vi "plotUpdate.vi"(6 "robotPosition":T2, 8 "plotPoints":cluster{dbl, dbl}[](array[cluster]), 11 "Image":T1) -> (3 "imageOut":T1)   [LabVIEW 2015]
uses:
  <vilib>/vision/Image Controls.llb/IMAQ Image.ctl
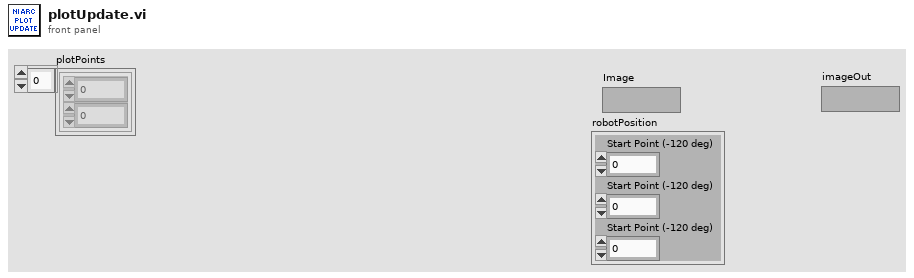
[diagram p1: front panel]
types:
  T1 = typedef "IMAQ Image.ctl" = refnum<image>
  T2 = cluster{"Start Point (-120 deg)":dbl, "Start Point (-120 deg)":dbl, "Start Point (-120 deg)":dbl}
  T3 = cluster{"Start Point (-120 deg)":dbl, "Start Point (-120 deg)":dbl}
  T4 = cluster{"Start Point (-120 deg)":dbl, "Start Point (-120 deg)":dbl, "Start Point (-120 deg)":dbl, "Start Point (-120 deg)":dbl}
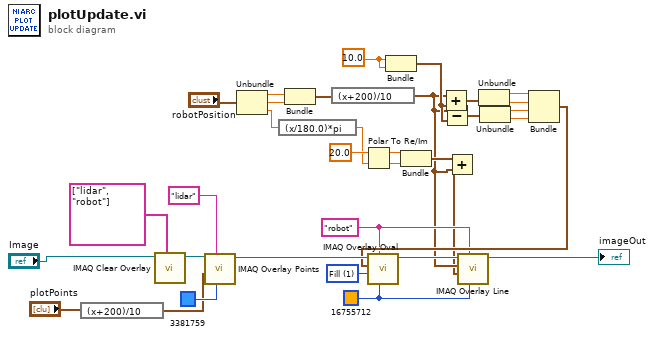
[diagram p0: block diagram]
diagram:
  w13 = u32 1 items=["Frame", "Fill"] ("Drawing Mode (Frame)")
  w22 = 10.0 ("Start Point (-120 deg)")
  w10 = "robot" ("Group")
  w11 = u32 16755712 ("Color")
  n1 = expression code="(x+200)/10"("plotPoints") -> (w30:cluster{dbl, dbl}[])
  n2 = call "IMAQ Clear Overlay"("Groups"=string[] ["lidar", "robot"], "Image"="Image") -> ("Image Out"=w32:T1)  [unwired: 8 in, 1 out]
  n3 = call "IMAQ Overlay Points"("Color"=u32 3381759, "Group"="lidar", "Array of Points"=w30, "Image"=w32) -> ("Image Out"=w27:T1)  [unwired: 6 in, 1 out]
  n4 = Unbundle("robotPosition") -> ("Start Point (-120 deg)"=w25:dbl, "Start Point (-120 deg)"=w24:dbl, "Start Point (-120 deg)"=w8:dbl)
  n5 = expression code="(x/180.0)*pi" ("degrees to radians")(w8) -> (w7:dbl)
  n6 = Bundle("Start Point (-120 deg)"=w25, "Start Point (-120 deg)"=w24) -> (w23:T3)  [unwired: 1 in]
  n7 = expression code="(x+200)/10"(w23) -> (w3:T3)
  n8 = Polar To Re/Im(2:w7, 3:20.0 ("r")) -> (0:w6:dbl, 1:w5:dbl)
  n9 = Bundle("Start Point (-120 deg)"=w22, "Start Point (-120 deg)"=w22) -> (w21:T3)  [unwired: 1 in]
  n10 = Bundle(w5, w6) -> (w4:cluster{dbl, dbl})  [unwired: 1 in]
  n11 = Add(x=w3, y=w21) -> (x+y=w20:T3)
  n12 = Subtract(x=w3, y=w21) -> (x-y=w19:T3)
  n13 = Add(x=w4, y=w3) -> (x+y=w2:cluster{dbl, dbl})
  n14 = Unbundle(w20) -> ("Start Point (-120 deg)"=w18:dbl, "Start Point (-120 deg)"=w17:dbl)
  n15 = Unbundle(w19) -> ("Start Point (-120 deg)"=w16:dbl, "Start Point (-120 deg)"=w15:dbl)
  n16 = Bundle("Start Point (-120 deg)"=w18, "Start Point (-120 deg)"=w17, "Start Point (-120 deg)"=w16, "Start Point (-120 deg)"=w15) -> (w14:T4)  [unwired: 1 in]
  n17 = call "IMAQ Overlay Oval"("Color"=w11, "Group"=w10, "Drawing Mode (Frame)"=w13, "Bounding Rectangle"=w14, "Image"=w27) -> ("Image Out"=w12:T1)  [unwired: 5 in, 1 out]
  n18 = call "IMAQ Overlay Line"("Color"=w11, "Group"=w10, "End Point"=w2, "Start Point"=w3, "Image"=w12) -> ("Image Out"=→"imageOut":T1)  [unwired: 5 in, 1 out]
